vi "FTW-Message-Metadata-Update.vi"(0 "Message In":T2, 7 "Metadata":string, 11 "error in":errorcluster, 12 "Update Mode (0: Upsert)":T1) -> (4 "Message":T2, 15 "error out":errorcluster)   [LabVIEW 2013]
uses:
  FTW-Message.ctl
  JSON/FTW-JSON-UpdateMode.ctl
  JSON/FTW-JSON.lvclass
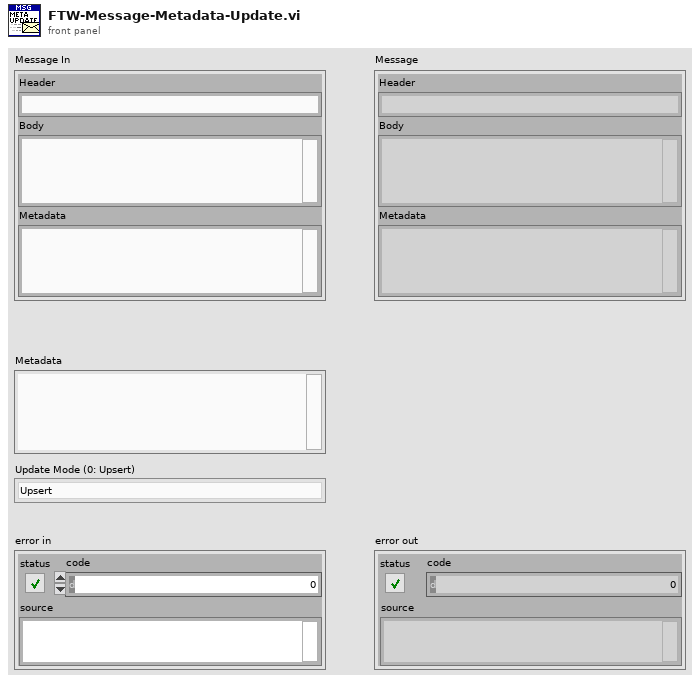
[diagram p1: front panel]
types:
  T1 = typedef "FTW-JSON.lvclass/FTW-JSON-UpdateMode.ctl" = enum16{"Upsert", "Update Only", "Insert Only"}
  T2 = typedef "FTW-Message.ctl" = cluster{"Header":string, "Body":string, "Metadata":string}
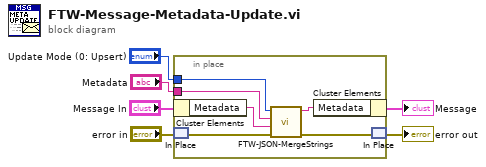
[diagram p0: block diagram]
diagram:
  n1 = in-place {
    in-place-border: "Update Mode (0: Upsert)" -> [w12]
    in-place-border: "Metadata" -> [w9]
    n2 = in-place-cluster #1("Message In") -> ("Metadata"=w10:string)
    n3 = in-place-match #2("error in") -> (w8:errorcluster)
    n4 = call "FTW-JSON-MergeStrings.vi"("error in (no error)"=w8, "Initial JSON String (\"\")"=w10, "JSON string to merge (\"\")"=w9, "Update Mode (0: Upsert)"=w12) -> ("error out"=w7:errorcluster, "Merged JSON String (UTF-8)"=w11:string)  [unwired: 6 in]
    n5 = in-place-cluster #1("Metadata"=w11) -> (→"Message":T2)
    n6 = in-place-match #2(w7) -> (→"error out":errorcluster)
  }
